vi "Read Result Channel GUID.vi"(8 "error in (no error)":errorcluster, 11 "WaveformCalculation in":refnum<class "WaveformCalculation.lvclass">) -> (0 "error out":errorcluster, 2 "Result Channel GUID":string, 3 "WaveformCalculation out":refnum<class "WaveformCalculation.lvclass">)   [LabVIEW 2015, in "WaveformCalculation.lvclass"]
uses:
  WaveformCalculation.lvclass
  WaveformCalculation.lvclass/WaveformCalculation.ctl
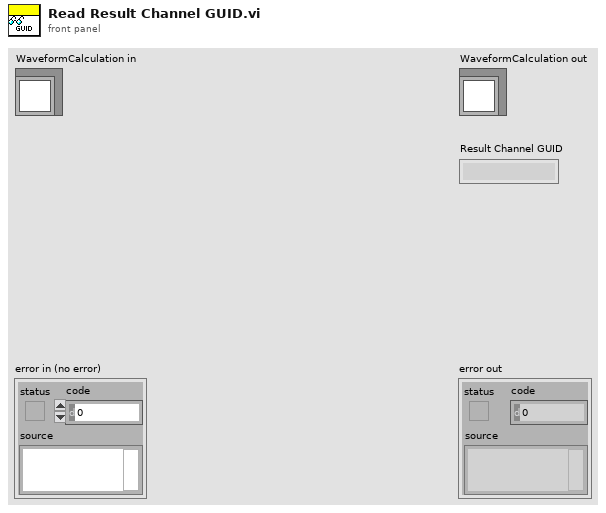
[diagram p1: front panel]
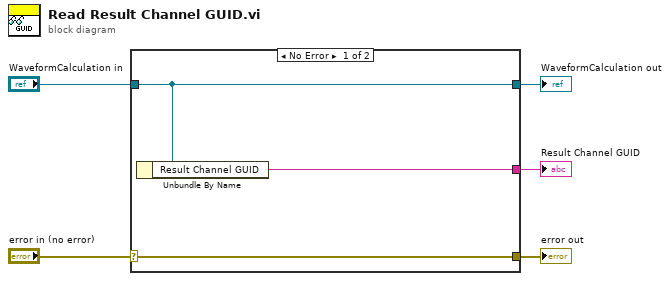
[diagram p0: block diagram]
diagram:
  n1 = case shown="No Error" "error in (no error)" {
    selector: "error in (no error)" -> [w8 w9]
    tunnel: [w8 w9] -> w4
    tunnel: [w7 w10] -> w2
    tunnel: "WaveformCalculation in" -> [w7 w10]
    tunnel: [w6 _] -> w1
    frame No Error {
      n2 = Unbundle By Name(w7) -> ("Result Channel GUID"=w6:string)
    }
    frame Error {
    }
  }
  "error out" <- w4
  "WaveformCalculation out" <- w2
  "Result Channel GUID" <- w1
